vi "Update_Progress_Bar-1.vi"(4 "error IN":errorcluster, 6 "[IN] Number of SubVI":i32, 7 "[IN] Tracking progress":refnum<vi>) -> (0 "error OUT":errorcluster, 3 "[OUT] Tracking progress":refnum<vi>)   [LabVIEW 2013]
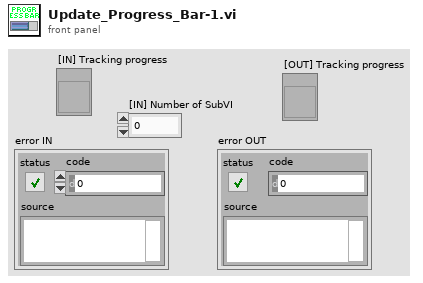
[diagram p1: front panel]
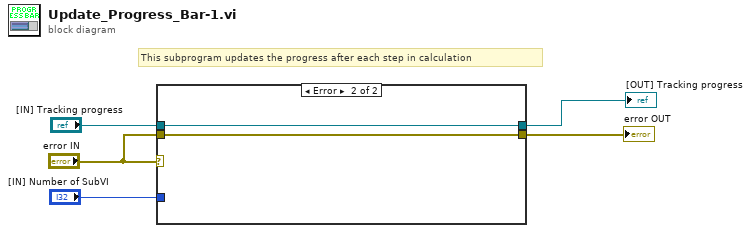
[diagram p0: block diagram]
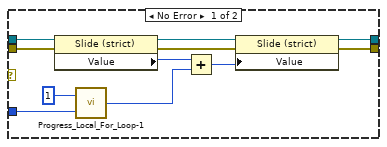
[diagram p2: hidden frame]
diagram:
  # "This subprogram updates the progress after each step in calculation"
  n1 = case shown="Error" "error IN" {
    tunnel: [w16 w18] -> w5
    tunnel: "error IN" -> [w14 w18]
    tunnel: "[IN] Tracking progress" -> [w13 w17]
    tunnel: "[IN] Number of SubVI" -> [w15 _]
    tunnel: [w6 w17] -> w1
    frame No Error {
      n2 = property on="Property Node" class="Slide (strict)"(reference=w13, error in=w14) -> (reference out=w11:refnum<vi>, error out=w12:errorcluster, "Value"=w9:u8)
      n3 = call "Progress_Local_For_Loop-1.vi"("[IN] Number of Frames"=w15, "[IN] Current Index"=1) -> ("[OUT] % progress"=w8:u8)
      n4 = Add(x=w9, y=w8) -> (x+y=w7:u8)
      n5 = property on="Property Node" class="Slide (strict)"(reference=w11, error in=w12, "Value"=w7) -> (reference out=w6:refnum<vi>, error out=w16:errorcluster)
    }
    frame Error {
    }
  }
  "error OUT" <- w5
  "[OUT] Tracking progress" <- w1
